vi "Ready Busy Status.vi"(8 "error in (no error)":errorcluster, 11 "Sync 2-Axis Stage Controller in":refnum<class "Sync 2-Axis Stage Controller.lvclass">) -> (0 "error out":errorcluster, 2 "Busy":bool, 3 "Sync 2-Axis Stage Controller out":refnum<class "Sync 2-Axis Stage Controller.lvclass">)   [LabVIEW 2022 SP3, in "Sync 2-Axis Stage Controller.lvclass"]
uses:
  Sync 2-Axis Stage Controller.lvclass
  Sync 2-Axis Stage Controller.lvclass/Sync 2-Axis Stage Controller.ctl
  Axis Objects/iMotion Controller/iMotion Controller.lvclass
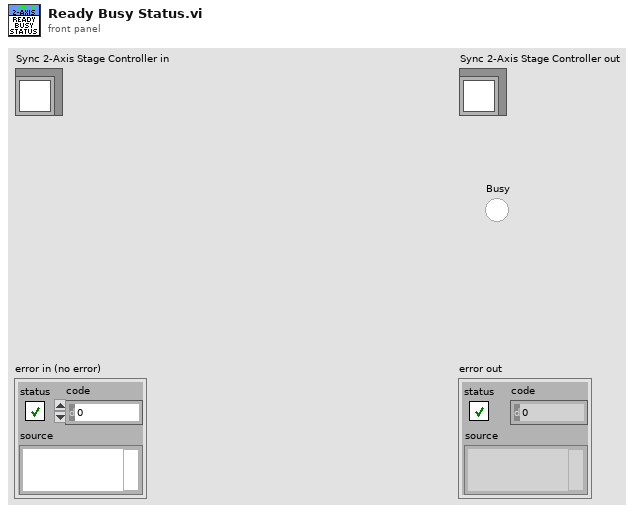
[diagram p1: front panel]
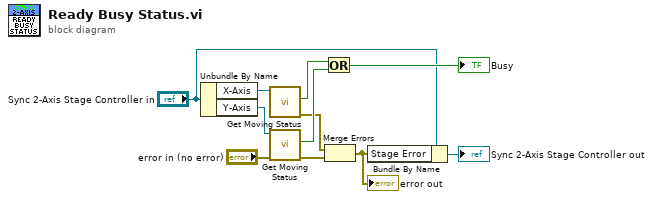
[diagram p0: block diagram]
diagram:
  n1 = Unbundle By Name("Sync 2-Axis Stage Controller in") -> ("X-Axis"=w11:refnum<class "iMotion Controller.lvclass">, "Y-Axis"=w10:refnum<class "iMotion Controller.lvclass">)
  n2 = call-dynamic "Get Moving Status.vi"("iMotion Controller in"=w11) -> ("error out"=w6:errorcluster, "Moving"=w8:bool)  [unwired: 8 in, 1 out]
  n3 = call-dynamic "Get Moving Status.vi"("error in (no error)"="error in (no error)", "iMotion Controller in"=w10) -> ("error out"=w5:errorcluster, "Moving"=w7:bool)  [unwired: 7 in, 1 out]
  n4 = Or(x=w8, y=w7) -> (x .or. y?=→"Busy":bool)
  n5 = Merge Errors(w6, w5) -> (w1:errorcluster)
  "error out" <- w1
  n6 = Bundle By Name(cluster="Sync 2-Axis Stage Controller in", "Stage Error"=w1) -> (→"Sync 2-Axis Stage Controller out":refnum<class "Sync 2-Axis Stage Controller.lvclass">)
